vi "CalcNumberOfPeriodPerPackage.vi"(0 "object in":refnum<class "Experiment.lvclass">, 5 "error in (no error)":errorcluster) -> (14 "object out":refnum<class "Experiment.lvclass">, 16 "Number Of Periods Per Package":dbl, 19 "error out":errorcluster)   [LabVIEW 2019, in "Experiment.lvclass"]
uses:
  Experiment.lvclass
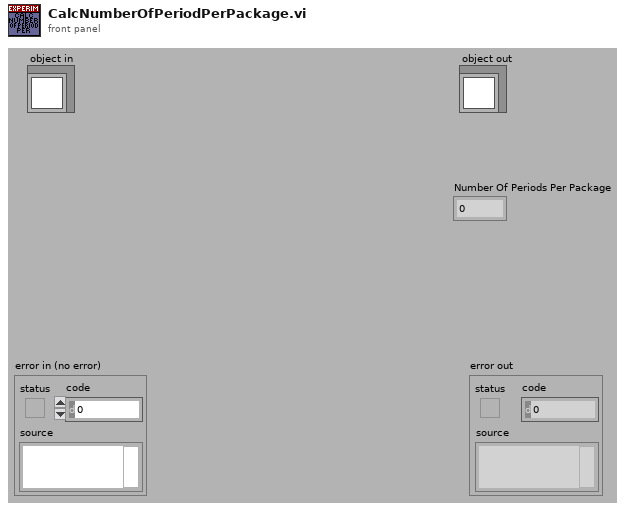
[diagram p1: front panel]
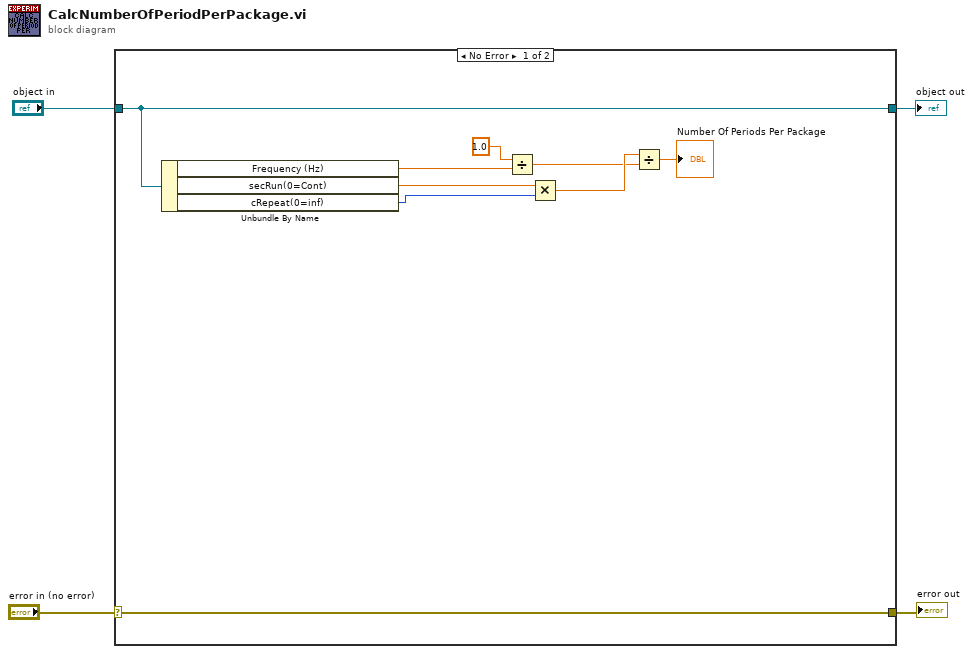
[diagram p0: block diagram]
diagram:
  n1 = case shown="No Error" "error in (no error)" {
    selector: "error in (no error)" -> [w13 w15]
    tunnel: [w13 w15] -> w3
    tunnel: [w12 w14] -> w1
    tunnel: "object in" -> [w12 w14]
    frame No Error {
      n2 = Unbundle By Name(w12) -> ("Frequency (Hz)"=w10:dbl, "secRun(0=Cont)"=w9:dbl, "cRepeat(0=inf)"=w8:i32)
      n3 = Divide(x=1.0, y=w10) -> (x/y=w6:dbl)
      n4 = Multiply(x=w9, y=w8) -> (x*y=w7:dbl)
      n5 = Divide(x=w7, y=w6) -> (x/y=→"Number Of Periods Per Package":dbl)
    }
    frame Error {
    }
  }
  "error out" <- w3
  "object out" <- w1
